vi "PDC On_Off.vi"(8 "error in (no error)":errorcluster {"code" format="%.0x"}, 10 "PDC (T:ON)":bool=TRUE, 11 "VISA Resource Name":refnum<visa-resource-name>) -> (0 "error out":errorcluster {"code" format="%.0x"}, 3 "VISA Resource Name Out":refnum<visa-resource-name>)   [LabVIEW 2012, in "Agilent ESG Series.lvlib"]
doc: "This VI is used to enable and disable the PDC communication standard.\nActivating the PDC personality sets up the internal hardware to generate a signal that follows the PDC protocol."
uses:
  <instrlib>/Agilent ESG Series/Agilent ESG Series.lvlib
panel:
  # "ON"
  # "OFF"
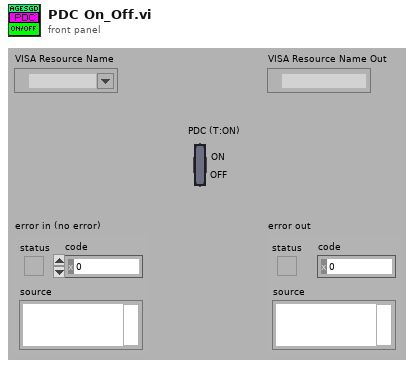
[diagram p1: front panel]
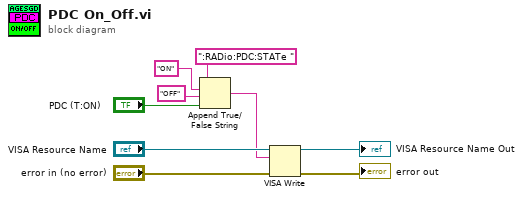
[diagram p0: block diagram]
diagram:
  n1 = Append True/False String(1:"PDC (T:ON)", 2:"OFF" ("false string"), 3:"ON" ("true string"), 4:":RADio:PDC:STATe ") -> (0:w2:string)
  n2 = VISA Write(VISA resource name="VISA Resource Name", write buffer=w2, error in (no error)="error in (no error)") -> (VISA resource name out=→"VISA Resource Name Out":refnum<visa-resource-name>, error out=→"error out":errorcluster)  [unwired: 1 out]
